vi "Make Integer List.vi"(8 "Error In":errorcluster, 9 "Start":i32, 10 "No. of elements":i32) -> (0 "Error Out":errorcluster, 1 "Integers Out":i32[](array[numeric]))   [LabVIEW 2017]
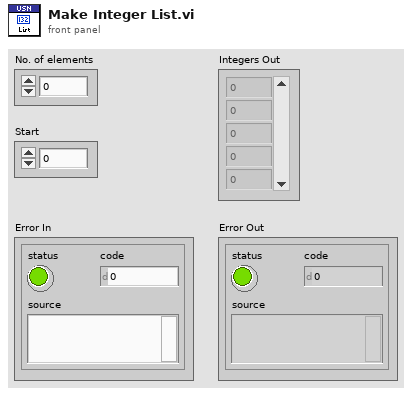
[diagram p1: front panel]
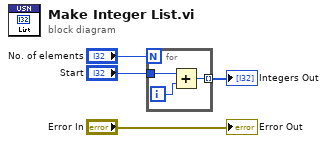
[diagram p0: block diagram]
diagram:
  n1 = for {
    N: "No. of elements" -> [_]
    tunnel: "Start" -> [w7]
    tunnel: [w5] -> w4 mode=indexing
    i -> [w6]
    n2 = Add(x=w7, y=w6) -> (x+y=w5:i32)
  }
  "Integers Out" <- w4
  "Error Out" <- "Error In"
